vi "GetTopicNode_etc.vi"(0 "node":string, 1 "Definitions":T4={"Topic"="/robot/head/command_head_nod", "Type"="std_msgs/Bool", "Action"=enum."Publisher", "Update (ms)"=1, "write queue"=1}) -> (2 "Server":T1={"vi name"="", "VI Refnum"=refnum, "queue"=refnum, "ROS"={"topic port"=0, "Node"="", "topic"="", "type"="", "node port"=0, "error "={"status"=FALSE, "code"=0, "source"=""}, "Direction"=enum."Node", "APIs"=[], "Update (ms)"=1, "write queue"=1}, "notifier"=refnum}, 3 "Already running?":bool, 4 "ROS":T2={"topic port"=0, "Node"="", "topic"="", "type"="", "node port"=0, "error "={"status"=FALSE, "code"=0, "source"=""}, "Direction"=enum."Node", "APIs"=[], "Update (ms)"=1, "write queue"=1})   [LabVIEW 2010]
uses:
  _ROSControl.ctl
  _ROSDirection.ctl
  Console/Servers/ServerSubs/TopicDef.ctl
  Console/Servers/ServerSubs/ServoInfo.ctl
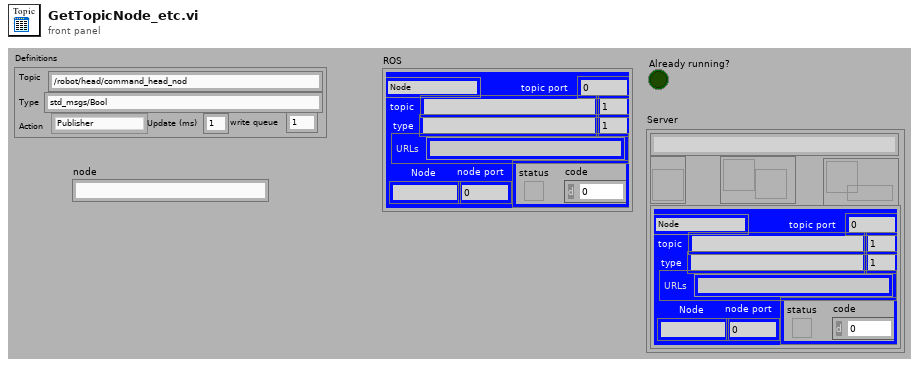
[diagram p1: front panel]
types:
  T1 = typedef "ServoInfo.ctl" = cluster{"vi name":string, "VI Refnum":refnum<vi>, "queue":refnum<queue>, "ROS":T2, "notifier":refnum<notifier>}
  T2 = typedef "_ROSControl.ctl" = cluster{"topic port":u16, "Node":string, "topic":string, "type":string, "node port":u32, "error ":errorcluster, "Direction":T3, "APIs":string[], "Update (ms)":u16, "write queue":u16}
  T3 = typedef "_ROSDirection.ctl" = enum16{"Node", "Publisher", "Subscriber", "Service Client"}
  T4 = typedef "TopicDef.ctl" = cluster{"Topic":string, "Type":string, "Action":T3, "Update (ms)":u16, "write queue":u16}
  T5 = enum16{"Get Nodes", "Start Nodes", "Reset Nodes"}
  T6 = cluster{"Topic":string, "Type":string, "Action":T3}
  T7 = cluster{"topic":string, "type":string, "Direction":T3}
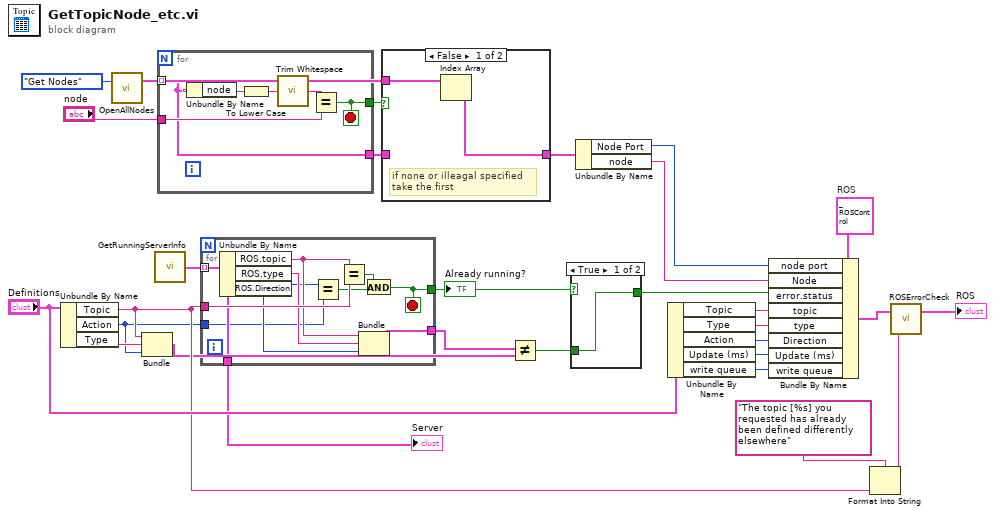
[diagram p0: block diagram]
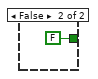
[diagram p2: hidden frame]
diagram:
  w20 = T2 {"topic port"=0, "Node"="", "topic"="", "type"="", "node port"=0, "error "={"status"=FALSE, "code"=0, "source"=""}, "Direction"=enum."Node", "APIs"=[], "Update (ms)"=0, "write queue"=0}  # ROS
  n1 = Unbundle By Name("Definitions") -> ("Topic"=w5:string, "Action"=w4:T3, "Type"=w6:string)
  n2 = call "OpenAllNodes.vi"("Task"=T5."Get Nodes") -> ("Nodes"=w9:cluster{"node":string, "Node Port":i32}[])  [unwired: 1 in]
  n3 = Bundle("Topic"=w5, "Type"=w6, "Action"=w4) -> (w3:T6)  [unwired: 1 in]
  n4 = call "GetRunningServerInfo.vi"() -> ("servers"=w13:T1[])  [unwired: 2 in, 2 out]
  n5 = for {
    tunnel: "node" -> [w33]
    tunnel: [w32] -> w26
    tunnel: [w30] -> w25
    tunnel: w9 -> [w30] mode=indexing
    stop <- w32 stop-if-true
    n6 = Unbundle By Name(w30) -> ("node"=w31:string)
    n7 = To Lower Case(string=w31) -> (all lower case string=w35:string)
    n8 = call <vilib>:"Trim Whitespace.vi"("string"=w35) -> ("trimmed string"=w34:string)  [unwired: 1 in]
    n9 = Equal?(x=w34, y=w33) -> (x = y?=w32:bool)
  }
  n10 = for {
    tunnel: w5 -> [w45]
    tunnel: [w36] -> w19
    tunnel: [w44] -> w15
    tunnel: w13 -> [w43] mode=indexing
    tunnel: [w43] -> w11
    tunnel: w4 -> [w39]
    stop <- w36 stop-if-true
    n11 = Unbundle By Name(w43) -> ("ROS.topic"=w42:string, "ROS.type"=w41:string, "ROS.Direction"=w40:T3)
    n12 = Equal?(x=w40, y=w39) -> (x = y?=w38:bool)
    n13 = Equal?(x=w42, y=w45) -> (x = y?=w37:bool)
    n14 = Bundle("topic"=w42, "type"=w41, "Direction"=w40) -> (w44:T7)  [unwired: 1 in]
    n15 = And(x=w37, y=w38) -> (x .and. y?=w36:bool)
  }
  "Already running?" <- w19
  "Server" <- w11
  n16 = case shown="False" w26 {
    tunnel: [w46 w48] -> w10
    tunnel: w25 -> [_ w48]
    tunnel: w9 -> [w47 _]
    frame False {
      # "if none or illeagal specified\ntake the first"
      n17 = Index Array(array=w47) -> (element=w46:cluster{"node":string, "Node Port":i32})  [unwired: 1 in]
    }
    frame True {
    }
  }
  n18 = Not Equal?(x=w15, y=w3) -> (x != y?=w14:bool)
  n19 = case shown="True" w19 {
    tunnel: [w49 FALSE] -> w28
    tunnel: w14 -> [w49 _]
    frame True {
    }
    frame False {
    }
  }
  n20 = Unbundle By Name(w10) -> ("Node Port"=w8:i32, "node"=w24:string)
  n21 = Unbundle By Name("Definitions") -> ("Topic"=w18:string, "Type"=w17:string, "Action"=w16:T3, "Update (ms)"=w2:u16, "write queue"=w1:u16)
  n22 = Bundle By Name(cluster=w20, "node port"=w8, "Node"=w24, "error.status"=w28, "topic"=w18, "type"=w17, "Direction"=w16, "Update (ms)"=w2, "write queue"=w1) -> (w23:T2)
  n23 = Format Into String(format string="The topic [%s] you requested has already been defined differently elsewhere" ("message"), w5) -> (resulting string=w21:string)  [unwired: 2 in, 1 out]
  n24 = call "ROSErrorCheck.vi"("message"=w21, "ROS in"=w23) -> ("ROS out"=→"ROS":T2)  [unwired: 1 in]
